vi "Trigger_Global.vi"() -> ()   [LabVIEW 2018]
panel:
  in  "Trigger":bool
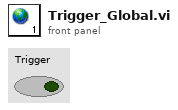
[diagram p1: front panel]
diagram:
